vi "Add Message Channel.vi"(8 "error in (no error)":errorcluster, 10 "Message Name":string, 11 "Message Group in":u64) -> (0 "error out":errorcluster, 1 "Message out":T1 format="%.0x", 3 "Message Group out":T1 format="%.0x")   [LabVIEW 2018, in "Instrument Addon Scripting API.lvlib"]
uses:
  Instrument Addon Scripting API.lvlib
  <vilib>/NI Veristand/Custom Device API/Custom Device Item Ref.ctl
  Addon/Addon Shared/SubVIs/Constants.vi
  Addon/Addon Shared/Instrument Addon Shared.lvlib
  <vilib>/NI Veristand/Custom Device API/Custom Device API.lvlib
  <vilib>/NI VeriStand/Custom Device Tools/Custom Device Utility Library/Custom Device Utility Library.lvlib
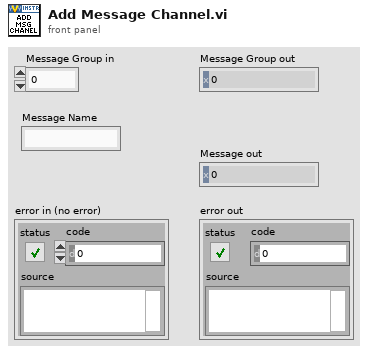
[diagram p1: front panel]
types:
  T1 = typedef "Custom Device API.lvlib/Custom Device Item Ref.ctl" = u64
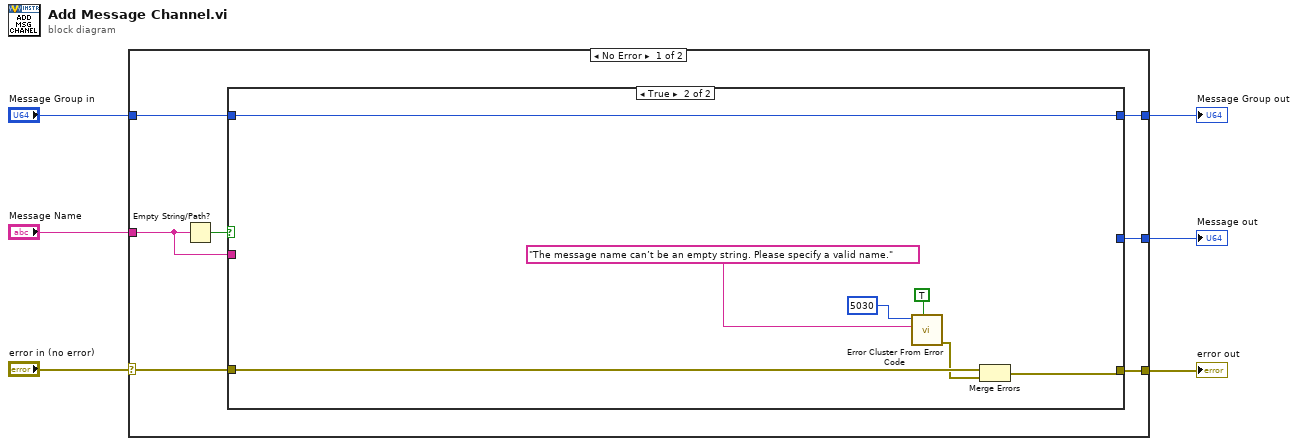
[diagram p0: block diagram]
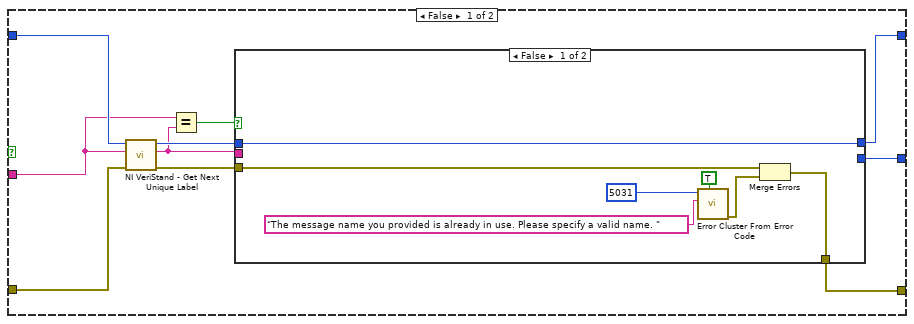
[diagram p2: hidden frame]
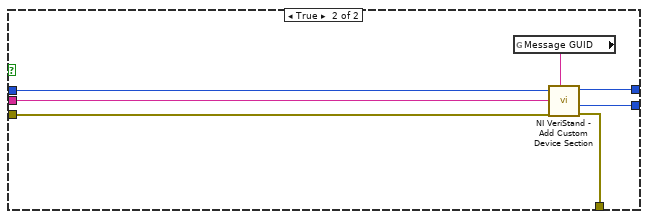
[diagram p3: hidden frame]
diagram:
  n1 = case shown="No Error" "error in (no error)" {
    selector: "error in (no error)" -> [w9 w46]
    tunnel: [w13 _] -> w6
    tunnel: [w12 w46] -> w5
    tunnel: [w11 w45] -> w4
    tunnel: "Message Name" -> [w7 _]
    tunnel: "Message Group in" -> [w10 w45]
    frame No Error {
      n2 = Empty String/Path?(string/path=w7) -> (empty?=w8:bool)
      n3 = case shown="True" w8 {
        tunnel: [w23 _] -> w13
        tunnel: [w22 w42] -> w12
        tunnel: [w21 w44] -> w11
        tunnel: w10 -> [w18 w44]
        tunnel: w9 -> [w17 w43]
        tunnel: w7 -> [w15 _]
        frame False {
          n4 = call <vilib>:"NI VeriStand - Get Next Unique Label.vi"("error in (no error)"=w17, "Label"=w15, "Parent Ref in"=w18) -> ("error out"=w20:errorcluster, "Label out"=w14:string, "Parent Ref dup"=w19:T1)  [unwired: 5 in, 1 out]
          n5 = Equal?(x=w15, y=w14) -> (x = y?=w16:bool)
          n6 = case shown="False" w16 {
            tunnel: [_ w37] -> w23
            tunnel: [w29 w36] -> w22
            tunnel: [w30 w34] -> w21
            tunnel: w20 -> [w28 w33]
            tunnel: w19 -> [w30 w32]
            tunnel: w14 -> [_ w31]
            frame False {
              n7 = call <vilib>:"Error Cluster From Error Code.vi"("show call chain? (False)"=TRUE, "error message (\"\")"="The message name you provided is already in use. Please specify a valid name. " ("error message (\"\")"), "error code (0)"=5031) -> ("error out"=w27:errorcluster)  [unwired: 6 in]
              n8 = Merge Errors(w28, w27) -> (w29:errorcluster)
            }
            frame True {
              n9 = global read "Constants.vi" "Message GUID"() -> (w35:string)
              n10 = call <vilib>:"NI VeriStand - Add Custom Device Section.vi"("GUID (Default Section)"=w35, "error in (no error)"=w33, "Section Name"=w31, "Parent Ref in"=w32) -> ("error out"=w36:errorcluster, "Section Ptr"=w37:T1, "Parent Ref out"=w34:T1)  [unwired: 4 in, 1 out]
            }
          }
        }
        frame True {
          n11 = call <vilib>:"Error Cluster From Error Code.vi"("show call chain? (False)"=TRUE, "error message (\"\")"="The message name can’t be an empty string. Please specify a valid name." ("error message (\"\")"), "error code (0)"=5030) -> ("error out"=w39:errorcluster)  [unwired: 6 in]
          n12 = Merge Errors(w43, w39) -> (w42:errorcluster)
        }
      }
    }
    frame Error {
    }
  }
  "Message out" <- w6
  "error out" <- w5
  "Message Group out" <- w4
